vi "eventSummaryState.vi"(8 "error in (no error)":errorcluster, 11 "Publisher in":refnum<class "Publisher.lvclass">) -> (0 "error out":errorcluster, 3 "Publisher out":refnum<class "Publisher.lvclass">)   [LabVIEW 2016, in "Publisher.lvclass"]
uses:
  Publisher.lvclass
  Publisher.lvclass/Publisher.ctl
  Communicator/Communicator/Communicator.lvclass
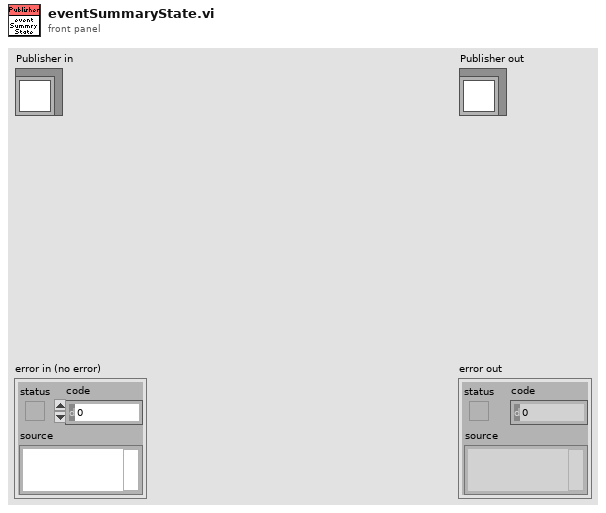
[diagram p1: front panel]
types:
  T1 = typedef "M1M3SupportTopics.lvlib/EventSummaryState.ctl" = cluster{"Timestamp":T2, "SummaryStates":T3}
  T2 = typedef "M1M3SupportTopics.lvlib/Timestamp.ctl" = dbl
  T3 = typedef "M1M3SupportTopics.lvlib/SummaryStates.ctl" = enum16{"OfflineState", "StandbyState", "DisabledState", "EnabledState", "FaultState"}
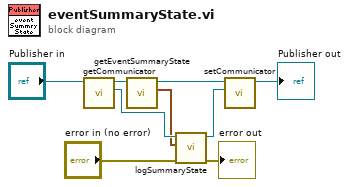
[diagram p0: block diagram]
diagram:
  n1 = call "getCommunicator.vi"("Publisher in"="Publisher in") -> ("Communicator"=w7:refnum<class "Communicator.lvclass">, "Publisher out"=w8:refnum<class "Publisher.lvclass">)  [unwired: 9 in]
  n2 = call "getEventSummaryState.vi"("Publisher in"=w8) -> ("EventSummaryState"=w6:T1, "Publisher out"=w4:refnum<class "Publisher.lvclass">)  [unwired: 9 in]
  n3 = call-dynamic "logSummaryState.vi"("error in (no error)"="error in (no error)", "EventSummaryState"=w6, "Communicator in"=w7) -> ("error out"=→"error out":errorcluster, "Communicator out"=w5:refnum<class "Communicator.lvclass">)  [unwired: 7 in]
  n4 = call "setCommunicator.vi"("Communicator"=w5, "Publisher in"=w4) -> ("Publisher out"=→"Publisher out":refnum<class "Publisher.lvclass">)  [unwired: 9 in]
